vi "Read All Dependencies Properties.vi"(8 "Error In":errorcluster, 11 "Custom Device .NET Ref In":refnum<k24>) -> (0 "Error Out":errorcluster, 2 "All Dependencies Properties":T1[](array[typedef]), 3 "Custom Device .NET Ref Out":refnum<k24>)   [LabVIEW 2015, in "VeriStand Custom Device XML Parser.lvlib"]
doc: "Reads and returns the properties of all dependencies of the custom device"
uses:
  VeriStand Custom Device XML Parser.lvlib
  XML Controls/Dependencies Properties.ctl
  XML Controls/Path Cluster.ctl
  XML Controls/Supported Targets.ctl
  NationalInstruments.VeriStand.XMLReader
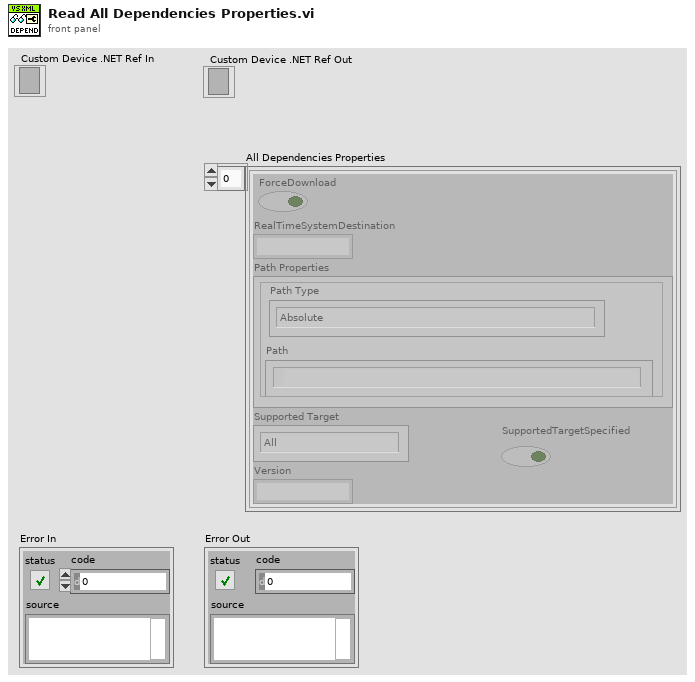
[diagram p1: front panel]
types:
  T1 = typedef "VeriStand Custom Device XML Parser.lvlib/Dependencies Properties.ctl" = cluster{"ForceDownload":bool, "RealTimeSystemDestination":string, "Path Properties":T2, "Supported Target":T3, "Version":string, "SupportedTargetSpecified":bool}
  T2 = typedef "VeriStand Custom Device XML Parser.lvlib/Path Cluster.ctl" = cluster{"Path":path, "Path Type":enum16{"Absolute", "To Base", "To Common Doc Dir", "To Application Data Dir"}}
  T3 = typedef "VeriStand Custom Device XML Parser.lvlib/Supported Targets.ctl" = enum16{"All", "Pharlap", "VxWorks", "Windows", "Linux_32_ARM", "Linux_x64", "PharlapWindows", "PharlapVxWorks", "VxWorksWindows"}
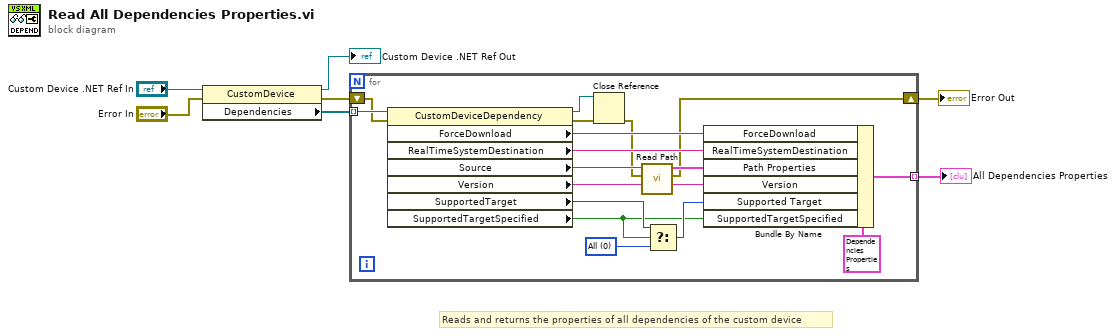
[diagram p0: block diagram]
diagram:
  # "Reads and returns the properties of all dependencies of the custom device"
  n1 = property class="CustomDevice"(reference="Custom Device .NET Ref In", error in="Error In") -> (reference out=→"Custom Device .NET Ref Out":refnum<k24>, error out=w4:errorcluster, "Dependencies"=w5:refnum<k24>[])
  n2 = for {
    tunnel: w5 -> [w24] mode=indexing
    shift-right: [w15] -> w6
    shift-left: w4 -> [w13]
    tunnel: [w14] -> w7 mode=indexing
    w10 = 0 items=["All", "Pharlap", "VxWorks", "Windows", "Linux_32_ARM", "Linux_x64", "PharlapWindows", "PharlapVxWorks", "VxWorksWindows"] ("SupportedTarget")
    n3 = property class="CustomDeviceDependency"(reference=w24, error in=w13) -> (reference out=w17:refnum<k24>, error out=w18:errorcluster, "ForceDownload"=w21:bool, "RealTimeSystemDestination"=w20:string, "Source"=w23:refnum<k24>, "Version"=w12:string, "SupportedTarget"=w11:i32, "SupportedTargetSpecified"=w8:bool)
    n4 = Close Reference(reference=w17, error in (no error)=w18) -> (error out=w16:errorcluster)
    n5 = call "Read Path.vi"("Error In"=w16, "Path .NET Ref"=w23) -> ("Error Out"=w15:errorcluster, "Path Properties"=w19:T2)  [unwired: 8 in]
    n6 = Select(t=w11, s=w8, f=w10) -> (s? t:f=w9:i32)
    n7 = Bundle By Name(cluster=T1 {"ForceDownload"=FALSE, "RealTimeSystemDestination"="", "Path Properties"={"Path"=path "", "Path Type"=enum."Absolute"}, "Supported Target"=enum."All", "Version"="", "SupportedTargetSpecified"=FALSE} ("output cluster"), "ForceDownload"=w21, "RealTimeSystemDestination"=w20, "Path Properties"=w19, "Version"=w12, "Supported Target"=w9, "SupportedTargetSpecified"=w8) -> (w14:T1)
  }
  "All Dependencies Properties" <- w7
  "Error Out" <- w6
